vi "KafkaStream_Read.vi"(0 "Consumer Handle":string, 5 "Group Name":string, 7 "Read Type":T1, 9 "Channel Names":string[](array[string]), 11 "error in (no error)":errorcluster) -> (1 "Property Names":string[][](array[string]), 3 "Property Values":variant[][](array[variant]), 4 "Consumer Handle Out":string, 6 "Group Name Out":string, 10 "Channel Names Out":string[](array[string]), 14 "Waveforms":waveform(dbl)[](array[waveform]), 15 "error out":errorcluster)   [LabVIEW 2019]
uses:
  support/_readType.ctl
panel:
  in  "Offset":i64
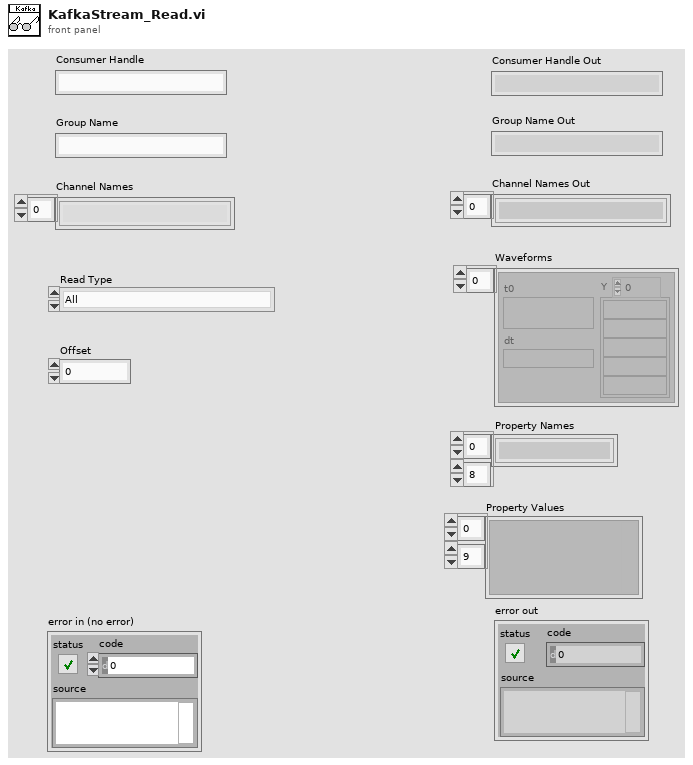
[diagram p1: front panel]
types:
  T1 = typedef "_readType.ctl" = enum16{"All", "Real-time", "Start Offset"}
  T2 = typedef "KafkaConsumerEvent.ctl" = cluster{"Payload":string, "Key":string, "MsgLen":u64, "Offset":i64, "Time Stamp":i64, "TS Name":string}
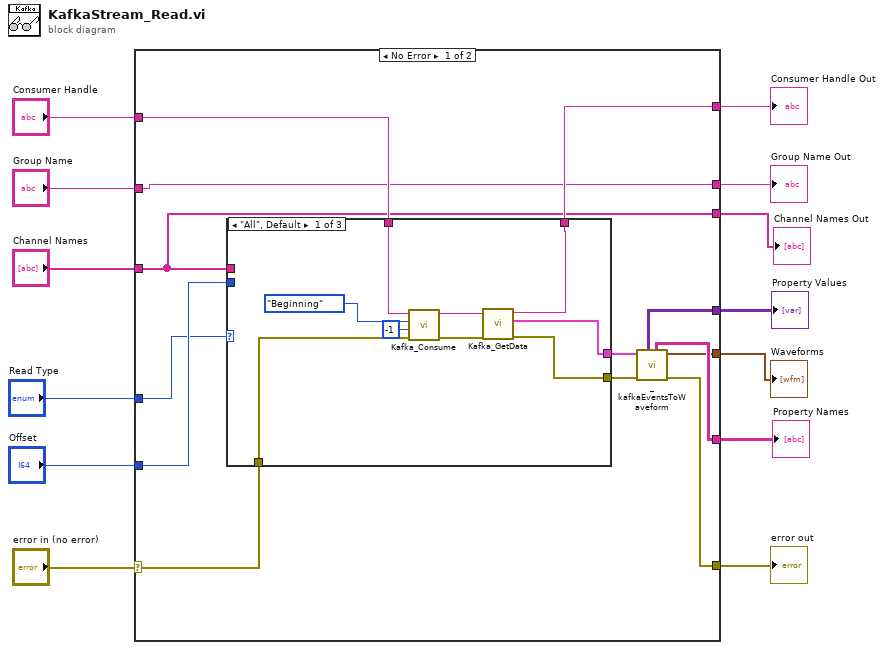
[diagram p0: block diagram]
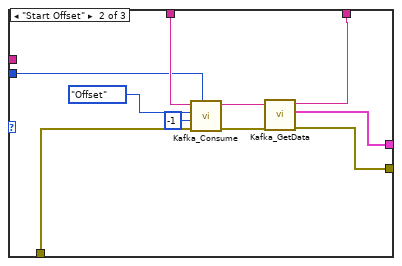
[diagram p2: hidden frame]
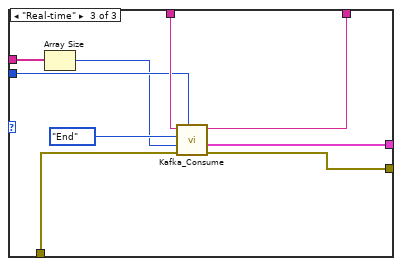
[diagram p3: hidden frame]
diagram:
  n1 = case shown="No Error" "error in (no error)" {
    selector: "error in (no error)" -> [w24 w55]
    tunnel: "Channel Names" -> [w14 _]
    tunnel: "Read Type" -> [w23 _]
    tunnel: "Consumer Handle" -> [w26 w56]
    tunnel: "Offset" -> [w25 _]
    tunnel: [w22 w56] -> w8
    tunnel: [w19 w55] -> w7
    tunnel: [w18 _] -> w6
    tunnel: [w17 _] -> w5
    tunnel: [w16 _] -> w4
    tunnel: "Group Name" -> [w15 _]
    tunnel: [w15 _] -> w2
    tunnel: [w14 _] -> w1
    frame No Error {
      n2 = case shown="\"All\", Default" w23 {
        tunnel: w26 -> [w35 w45 w54]
        tunnel: w25 -> [_ w36 w53]
        tunnel: w24 -> [w32 w42 w52]
        tunnel: w14 -> [_ _ w50]
        tunnel: [w29 w39 w46] -> w21
        tunnel: [w33 w43 w48] -> w22
        tunnel: [w30 w40 w47] -> w20
        frame "All", Default {
          n3 = call "Kafka_Consume.vi"("error in (no error)"=w32, "Max Events"=i64 -1, "Kafka Offset"=enum16{"Beginning", "End", "Offset"}."Beginning", "Consumer Handle"=w35) -> ("error out"=w31:errorcluster, "Consumer Handle"=w34:string)  [unwired: 4 in, 2 out]
          n4 = call "Kafka_GetData.vi"("error in (no error)"=w31, "Consumer Handle"=w34) -> ("error out"=w30:errorcluster, "Events"=w29:T2[], "Consumer Handle"=w33:string)  [unwired: 7 in]
        }
        frame "Start Offset" {
          n5 = call "Kafka_Consume.vi"("Offset Index"=w36, "error in (no error)"=w42, "Max Events"=i64 -1, "Kafka Offset"=enum16{"Beginning", "End", "Offset"}."Offset", "Consumer Handle"=w45) -> ("error out"=w41:errorcluster, "Consumer Handle"=w44:string)  [unwired: 3 in, 2 out]
          n6 = call "Kafka_GetData.vi"("error in (no error)"=w41, "Consumer Handle"=w44) -> ("error out"=w40:errorcluster, "Events"=w39:T2[], "Consumer Handle"=w43:string)  [unwired: 7 in]
        }
        frame "Real-time" {
          n7 = Array Size(array=w50) -> (size(s)=w49:i32)
          n8 = call "Kafka_Consume.vi"("Offset Index"=w53, "error in (no error)"=w52, "Max Events"=w49, "Kafka Offset"=enum16{"Beginning", "End", "Offset"}."End", "Consumer Handle"=w54) -> ("error out"=w47:errorcluster, "Kafka Events"=w46:T2[], "Consumer Handle"=w48:string)  [unwired: 3 in, 1 out]
        }
      }
      n9 = call "_kafkaEventsToWaveform.vi"("error"=w20, "Kafka Events"=w21) -> ("error out"=w19:errorcluster, "Waveforms"=w16:waveform(dbl)[], "Names"=w17:string[][], "Values"=w18:variant[][])  [unwired: 6 in]
    }
    frame Error {
    }
  }
  "Group Name Out" <- w2
  "Consumer Handle Out" <- w8
  "Channel Names Out" <- w1
  "Waveforms" <- w4
  "error out" <- w7
  "Property Names" <- w5
  "Property Values" <- w6
